vi "MyG#G3Templ_GetClassAttributesToModify.vi"(0 "reference in":refnum<class "MyG#G3Templ.lvclass">, 3 "timeout in ms (-1)":i32=-1, 5 "error in (no error)":errorcluster) -> (14 "reference out":refnum<class "MyG#G3Templ.lvclass">, 15 "class attributes ref":T2, 16 "class attributes":T1, 17 "timeout":bool, 18 "created new":bool, 19 "error out":errorcluster)   [LabVIEW 2017, in "MyG#G3Templ.lvclass"]
doc: "This VI returns the attributes associated with this class or subclass object reference and places a lock on the object.\n\nIf the object is currently locked for modification by another method, 'Timeout' specifies how long the VI should wait to receive access to the object. The default value waits until the object becomes available.\n\nYou must use this class SetModifiedAttributes VI to set the object's data and release the lock."
uses:
  MyG#G3Templ.lvclass
  ClassAttributesRef.ctl
  protected/ClassAttributes.ctl
  MyG#G3Templ.lvclass/MyG#G3Templ.ctl
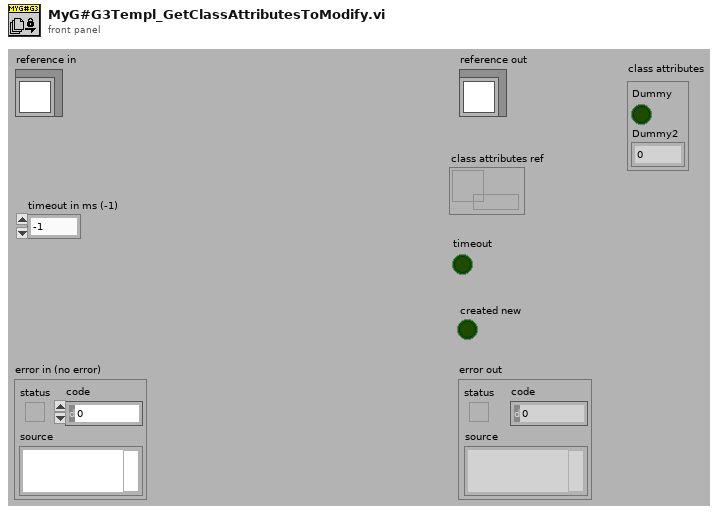
[diagram p1: front panel]
types:
  T1 = typedef "MyG#G3Templ.lvclass/ClassAttributes.ctl" = cluster{"Dummy":bool, "Dummy2":dbl}
  T2 = typedef "MyG#G3Templ.lvclass/ClassAttributesRef.ctl" = refnum<data-value>
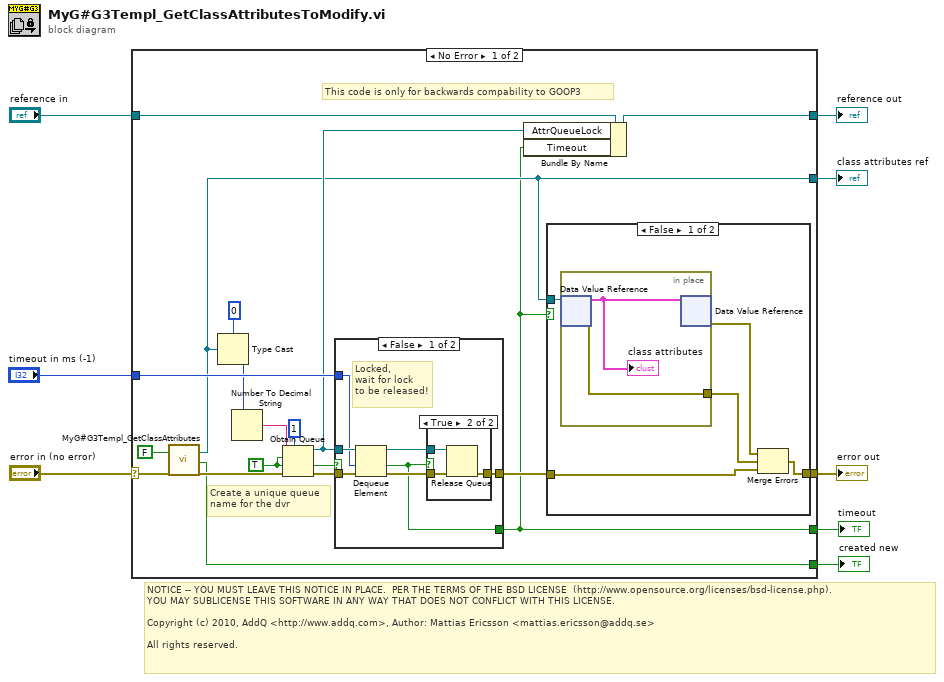
[diagram p0: block diagram]
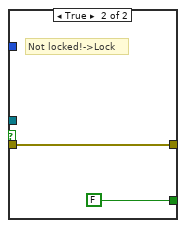
[diagram p3: hidden frame]
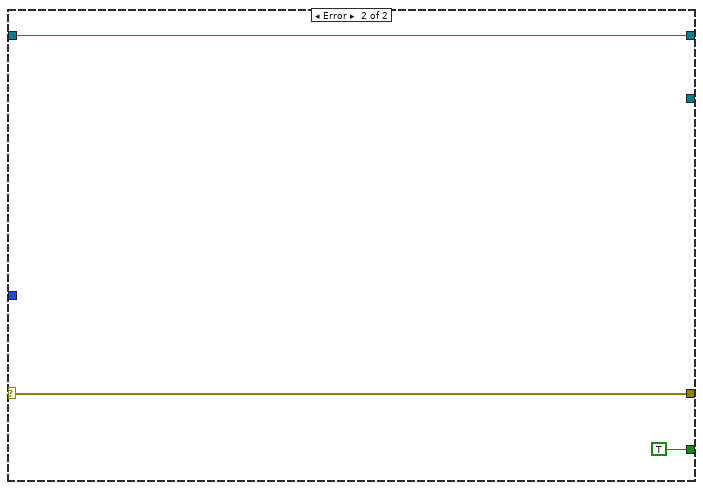
[diagram p5: hidden frame]
diagram:
  # "NOTICE -- YOU MUST LEAVE THIS NOTICE IN PLACE.  PER THE TERMS OF THE BSD LICENSE  (http://www.opensource.org/licenses/bsd-license.php).\nYOU MAY SUBLICENSE THIS SOFTWARE IN ANY WAY THAT DOES NOT CONFLICT WITH THIS LICENSE.\n\nCopyright (c) 2010, AddQ <http://www.addq.com>, Author: Mattias Ericsson <mattias.ericsson@addq.se>\n\nAll rights reserved."
  n1 = case shown="No Error" "error in (no error)" {
    selector: "error in (no error)" -> [w16 w51]
    tunnel: [w27 w51] -> w7
    tunnel: [w18 w50] -> w5
    tunnel: "reference in" -> [w19 w50]
    tunnel: [w13 _] -> w4
    tunnel: "timeout in ms (-1)" -> [w20 _]
    tunnel: [w10 TRUE ("status")] -> w2
    tunnel: [w9 _] -> w1
    frame No Error {
      w25 = TRUE ("create if not found? (T)")
      # "Create a unique queue\nname for the dvr"
      # "This code is only for backwards compability to GOOP3"
      n2 = call "MyG#G3Templ_GetClassAttributes.vi"("return data"=FALSE, "error in (no error)"=w16) -> ("class attributes ref"=w13:T2, "created new"=w9:bool, "error out"=w15:errorcluster)  [unwired: 13 in, 2 out]
      n3 = Type Cast(type=u32 0, x=w13) -> (*(type *) &x=w12:u32)
      n4 = Number To Decimal String(number=w12) -> (decimal integer string=w26:string)  [unwired: 1 in]
      n5 = Obtain Queue(max queue size (-1, unlimited)=1, name (unnamed)=w26, element data type=w25, create if not found? (T)=w25, error in (no error)=w15) -> (queue out=w17:refnum<queue>, created new?=w22:bool, error out=w23:errorcluster)
      n6 = case shown="False" w22 {
        tunnel: w23 -> [w32 w39]
        tunnel: [w31 w39] -> w21
        tunnel: w17 -> [w34 _]
        tunnel: w20 -> [w33 _]
        tunnel: [w28 FALSE ("status")] -> w10
        frame False {
          # "Locked,\nwait for lock\nto be released!"
          n7 = Dequeue Element(queue=w34, timeout in ms (-1)=w33, error in (no error)=w32) -> (queue out=w29:refnum<queue>, timed out?=w28:bool, error out=w30:errorcluster)  [unwired: 1 out]
          n8 = case shown="True" w28 {
            tunnel: [w35 w38] -> w31
            tunnel: w30 -> [w35 w37]
            tunnel: w29 -> [_ w36]
            frame False {
            }
            frame True {
              n9 = Release Queue(queue=w36, error in (no error)=w37) -> (error out=w38:errorcluster)  [unwired: 1 in, 2 out]
            }
          }
        }
        frame True {
          # "Not locked!->Lock"
        }
      }
      n10 = Bundle By Name(cluster=w19, "AttrQueueLock"=w17, "Timeout"=w10) -> (w18:refnum<class "MyG#G3Templ.lvclass">)
      n11 = case shown="False" w10 {
        tunnel: w13 -> [w45 _]
        tunnel: w21 -> [w44 w48]
        tunnel: [w41 w48] -> w27
        frame False {
          n12 = in-place {
            in-place-border: [w47] -> w43
            n13 = in-place-dvr #1(w45) -> (w46:T1, w47:errorcluster)
            "class attributes" <- w46
            n14 = in-place-dvr #1(w46) -> (w42:errorcluster)  [unwired: 1 out]
          }
          n15 = Merge Errors(w42, w43, w44) -> (w41:errorcluster)
        }
        frame True {
        }
      }
    }
    frame Error {
    }
  }
  "error out" <- w7
  "reference out" <- w5
  "class attributes ref" <- w4
  "timeout" <- w2
  "created new" <- w1
